vi "Reset.vi"(11 "direct handler in":refnum<class "Direct Handler.lvclass">) -> (2 "successful?":bool, 3 "direct handler out":refnum<class "Direct Handler.lvclass">)   [LabVIEW 2018, in "Logging.lvlib" / "Direct Handler.lvclass"]
uses:
  Direct Handler.lvclass
  formatting_handler_interface/Formatting Handler.lvclass
panel:
  # "Connector Pane"
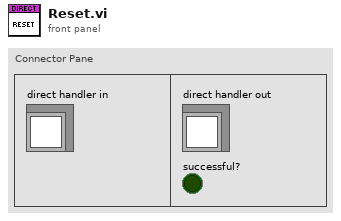
[diagram p1: front panel]
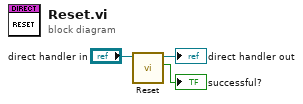
[diagram p0: block diagram]
diagram:
  n1 = call-parent "Reset.vi"("handler in"="direct handler in") -> ("successful?"=→"successful?":bool, "handler out"=→"direct handler out":refnum<class "Direct Handler.lvclass">)  [unwired: 9 in]
